vi "ReadDataFile_V2.vi"(6 "Channel Name Array Size":i32, 7 "Resolution":string, 8 "error in (no error)":errorcluster, 9 "Create CSV files?":bool, 10 "Channel Name Individual":string, 11 "DataFolder Path":path) -> (0 "error out":errorcluster, 2 "Current Measurements Individual":cluster{dbl[], dbl[]}, 3 "Voltage Measurements Individual":cluster{dbl[], dbl[]})   [LabVIEW 2019]
uses:
  <vilib>/Utility/file.llb/Write Delimited Spreadsheet (string).vi
panel:
  in  "Channel Names Array":string[](array[string])
  out "Voltage Measurements":cluster{dbl[], dbl[]}[](array[cluster])
  out "Current Measurements":cluster{dbl[], dbl[]}[](array[cluster])
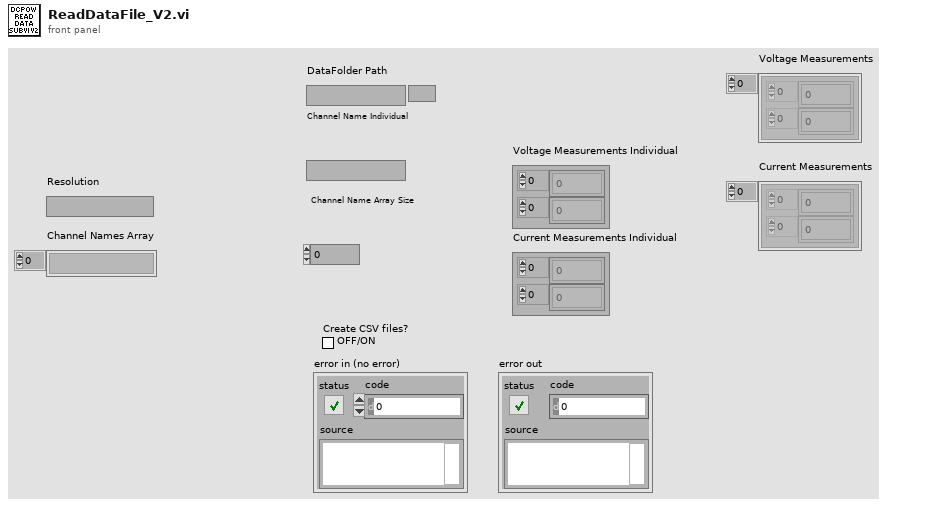
[diagram p1: front panel]
types:
  T1 = enum16{"big-endian, network order", "native, host order", "little-endian"}
  T2 = cluster{"Array of fetched data":dbl[][], string, i32[]}
  T3 = enum16{"open", "replace", "create", "open or create", "replace or create", "replace or create with confirmation"}
  T4 = cluster{"Array of fetched data":dbl[][], string, i32[]}[]
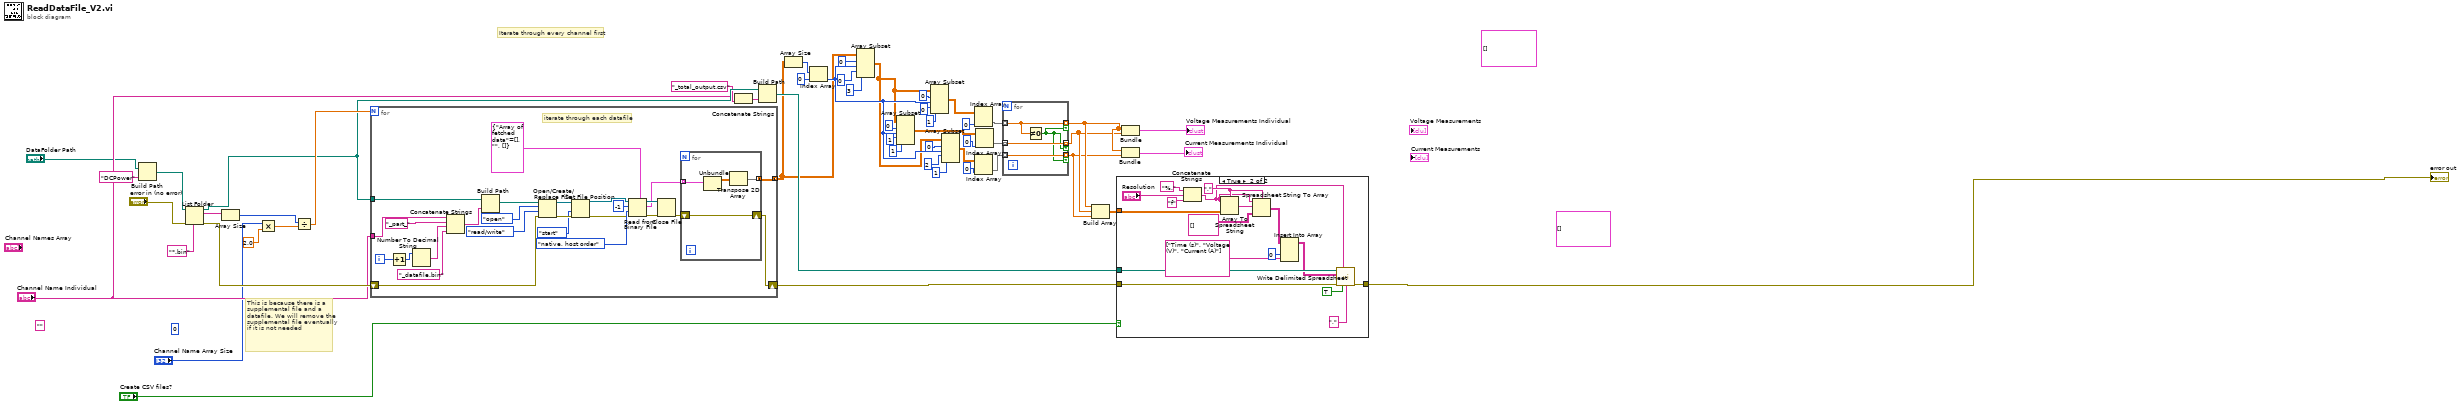
[diagram p0: block diagram]
diagram:
  (unwired) 0
  (unwired) ""
  (unwired) cluster{dbl[], dbl[]}[] []
  (unwired) cluster{dbl[], dbl[]}[] []
  # "Iterate through every channel first"
  # "This is because there is a supplemental file and a datafile. We will remove the supplemental file eventually if it is not needed"
  n1 = Build Path(base path="DataFolder Path", name or relative path="DCPower") -> (appended path=w1:path)
  n2 = List Folder(path=w1, pattern="*.bin", error in="error in (no error)") -> (path out=w48:path, filenames=w44:string[], error out=w50:errorcluster)  [unwired: 1 in, 1 out]
  n3 = Array Size(array=w44) -> (size(s)=w47:i32)
  n4 = Multiply(x="Channel Name Array Size", y=2.0) -> (x*y=w46:dbl)
  n5 = Divide(x=w47, y=w46) -> (x/y=w49:dbl)
  n6 = for {
    N: w49 -> [_]
    tunnel: "Channel Name Individual" -> [w78]
    tunnel: w48 -> [w74]
    shift-right: [w54] -> w36
    shift-left: w50 -> [w69]
    tunnel: [w53] -> w13 mode=concatenating
    i -> [w58]
    # "iterate through each datafile"
    n7 = Increment(x=w58) -> (x+1=w57:i32)
    n8 = Number To Decimal String(number=w57) -> (decimal integer string=w76:string)  [unwired: 1 in]
    n9 = Concatenate Strings(w78, "_part_" ("string"), w76, "_datafile.bin" ("string")) -> (w73:string)
    n10 = Build Path(base path=w74, name or relative path=w73) -> (appended path=w72:path)
    n11 = Open/Create/Replace File(file path (use dialog)=w72, error in=w69, operation (0:open)=T3."open", access (0:read/write)=enum16{"read/write", "read-only", "write-only"}."read/write") -> (refnum out=w62:refnum<file>, error out=w63:errorcluster)  [unwired: 2 in, 1 out]
    n12 = Set File Position(refnum=w62, from (0:start)=enum16{"start", "end", "current"}."start", error in=w63) -> (refnum out=w59:refnum<file>, error out=w60:errorcluster)  [unwired: 1 in]
    n13 = Read from Binary File(5:T2 {"Array of fetched data"=[], "", []} ("cluster"), 8:w60, 9:T1."native, host order" ("byte order (0:big-endian, network order)"), 10:-1 ("count (1)"), 11:w59) -> (0:w65:errorcluster, 2:w56:T4, 3:w64:refnum<file>)  [unwired: 1 in, 1 out]
    n14 = Close File(refnum=w64, error in=w65) -> (error out=w55:errorcluster)  [unwired: 1 out]
    n15 = for {
      tunnel: w56 -> [w82] mode=indexing
      tunnel: [w79] -> w53 mode=concatenating
      shift-right: [w81] -> w54
      shift-left: w55 -> [w81]
      n16 = Unbundle(w82) -> ("Array of fetched data"=w80:dbl[][])  [unwired: 2 out]
      n17 = Transpose 2D Array(2D array=w80) -> (transposed array=w79:dbl[][])
    }
  }
  n18 = Concatenate Strings("Channel Name Individual", "_total_output.csv" ("string")) -> (w39:string)
  n19 = Build Path(base path=w48, name or relative path=w39) -> (appended path=w37:path)
  n20 = Array Size(array=w13) -> (size(s)=w41:i32[])
  n21 = Index Array(array=w41, index=0) -> (element=w23:i32)
  n22 = Array Subset(array=w13, index (row)=0 ("index"), length (row)=w23, index (col)=0 ("index"), length (col)=3 ("length")) -> (w12:dbl[][])
  n23 = Array Subset(array=w12, index (row)=0 ("index"), length (row)=w23, index (col)=1 ("index"), length (col)=1 ("length")) -> (w21:dbl[][])
  n24 = Array Subset(array=w12, index (row)=0 ("index"), length (row)=w23, index (col)=0 ("index"), length (col)=1 ("length")) -> (w22:dbl[][])
  n25 = Array Subset(array=w12, index (row)=0 ("index"), length (row)=w23, index (col)=2 ("index"), length (col)=1 ("length")) -> (w20:dbl[][])
  n26 = Index Array(array=w22, index (col)=0 ("disabled index (col)")) -> (element=w16:dbl[])  [unwired: 1 in]
  n27 = Index Array(array=w20, index (col)=0 ("disabled index (col)")) -> (element=w14:dbl[])  [unwired: 1 in]
  n28 = Index Array(array=w21, index (col)=0 ("disabled index (col)")) -> (element=w15:dbl[])  [unwired: 1 in]
  n29 = for {
    tunnel: w16 -> [w83] mode=indexing
    tunnel: w15 -> [w86] mode=indexing
    tunnel: w14 -> [w85] mode=indexing
    tunnel: [w83] -> w11 mode=indexing if=w84
    tunnel: [w86] -> w10 mode=indexing if=w84
    tunnel: [w85] -> w9 mode=indexing if=w84
    n30 = Not Equal To 0?(x=w83) -> (x != 0?=w84:bool)
  }
  n31 = Build Array(w11, w10, w9) -> (w8:dbl[][])
  n32 = case shown="True" "Create CSV files?" {
    tunnel: w37 -> [_ w104]
    tunnel: w36 -> [w87 w103]
    tunnel: [w87 w102] -> w42
    tunnel: w8 -> [_ w96]
    frame False {
    }
    frame True {
      w100 = "," ("delimiter (Tab)")
      n33 = Concatenate Strings("%." ("string"), "Resolution", "f" ("string")) -> (w89:string)
      n34 = Array To Spreadsheet String(delimiter (Tab)=w100, array=w96, 3:w89) -> (spreadsheet string=w99:string)
      n35 = Spreadsheet String To Array(delimiter (Tab)=w100, format string=w89, spreadsheet string=w99, array type (2D Dbl)=string[][] []) -> (array=w95:string[][])
      n36 = Insert Into Array(array=w95, index (col)=0 ("disabled index (col)"), new element=string[] ["Time (s)", "Voltage (V)", "Current (A)"]) -> (w93:string[][])  [unwired: 1 in]
      n37 = call-poly <vilib>:"Write Delimited Spreadsheet.vi"("file path (dialog if empty)"=w104, "format (%s)"=w89, "2D data"=w93, "error in (no error)"=w103, "transpose? (no:F)"=TRUE, "delimiter (\\t)"="," ("delimiter (\\t)")) -> ("error out"=w102:errorcluster)  [unwired: 8 in, 1 out]
    }
  }
  "error out" <- w42
  n38 = Bundle(w11, w9) -> (→"Current Measurements Individual":cluster{dbl[], dbl[]})  [unwired: 1 in]
  n39 = Bundle(w11, w10) -> (→"Voltage Measurements Individual":cluster{dbl[], dbl[]})  [unwired: 1 in]
